vi "HFRR ADV v07.vi"() -> ()   [LabVIEW 2025] (continued)
1.7013246142177483, 1.7065972599989456, 1.7083548085926759, 1.7101123571864059, 1.7136274543738683, 1.7171425515613308, 1.722415197342526, 1.7153850029676008, 1.7101123571864059, 1.7101123571864059, 1.7276878431237184, 1.7171425515613308, 1.7171425515613308, 1.7259302945299884, 1.7259302945299884, 1.741748231873566, 1.7364755860923762, 1.7364755860923762, 1.739990683279836, 1.739990683279836, 1.7382331346861086, 1.7435057804672986, 1.7329604889049162, 1.7329604889049162, 1.7259302945299884, 1.7136274543738683, 1.7101123571864059, 1.7083548085926759, 1.7083548085926759, 1.7083548085926759, 1.7171425515613308, 1.7065972599989456, 1.6960519684365558, 1.6960519684365558, 1.6942944198428282, 1.697809517030288, 1.6960519684365558, 1.6960519684365558, 1.6942944198428282, 1.697809517030288, 1.6925368712490982, 1.6942944198428282, 1.6960519684365558, 1.6890217740616331, 1.6872642254679004, 1.6942944198428282, 1.6837491282804407, 1.6872642254679004, 1.6837491282804407, 1.6802340310929782, 1.6784764824992453, 1.6907793226553656, 1.6855066768741707, 1.6802340310929782, 1.6767189339055155, 1.6749613853117828, 1.6767189339055155, 1.681991579686708, 1.681991579686708, 1.6942944198428282, 1.6890217740616331, 1.6855066768741707, 1.6960519684365558, 1.6925368712490982, 1.6925368712490982, 1.697809517030288, 1.7101123571864059, 1.7083548085926759, 1.7083548085926759, 1.7136274543738683, 1.7189001001550634, 1.7259302945299884, 1.7276878431237184, 1.734718037498646, 1.7329604889049162, 1.7312029403111808, 1.7329604889049162, 1.7382331346861086, 1.734718037498646, 1.7329604889049162, 1.7312029403111808, 1.7329604889049162, 1.734718037498646, 1.739990683279836, 1.7435057804672986, 1.7435057804672986, 1.7470208776547638, 1.7487784262484938, 1.757566169217149, 1.7540510720296862, 1.7558086206234187, 1.771626557966999, 1.7645963635920765, 1.7645963635920765, 1.824353015778937, 1.884109667965795, 1.7997473354666966, 1.7839293981231163, 1.7856869467168466, 1.787444495310579, 1.792717141091774, 1.787444495310579, 1.7804143009356566, 1.782171849529389, 1.7804143009356566, 1.7786567523419266, 1.787444495310579, 1.776899203748194, 1.782171849529389, 1.776899203748194, 1.776899203748194, 1.7804143009356566, 1.787444495310579, 1.792717141091774, 1.7909595924980442, 1.7997473354666966, 1.8050199812478944, 1.8050199812478944, 1.8102926270290869, 1.8120501756228167, 1.8173228214040091, 1.8208379185914743, 1.824353015778937, 1.831383210153857, 1.833140758747592, 1.833140758747592, 1.8366558559350545, 1.8401709531225146, 1.833140758747592, 1.834898307341322, 1.8436860503099772, 1.8366558559350545, 1.8384134045287848, 1.8366558559350545, 1.8384134045287848, 1.8472011474974424, 1.8436860503099772, 1.8507162446849048, 1.8595039876535597, 1.8542313418723673, 1.8612615362472924, 1.866534182028485, 1.8682917306222173, 1.866534182028485, 1.8682917306222173, 1.866534182028485, 1.8682917306222173, 1.8718068278096776, 1.8770794735908725, 1.8700492792159473, 1.8700492792159473, 1.87532192499714, 1.884109667965795, 1.884109667965795, 1.8876247651532576, 1.8893823137469927, 1.8911398623407227, 1.8893823137469927, 1.8946549595281854, 1.898170056715645, 1.898170056715645, 1.8964125081219152, 1.8999276053093779, 1.9016851539031077, 1.9052002510905728, 1.9052002510905728, 1.912230445465498, 1.9069577996843026, 1.9052002510905728, 1.9069577996843026, 1.912230445465498, 1.9052002510905728, 1.9034427024968403, 1.9034427024968403, 1.9016851539031077, 1.9016851539031077, 1.9069577996843026, 1.9104728968717652, 1.912230445465498, 1.9175030912466904, 1.9210181884341528, 1.9210181884341528, 1.913987994059228, 1.9175030912466904, 1.9333210285902707, 1.9227757370278828, 1.9280483828090755, 1.935078577184003, 1.9368361257777331, 1.935078577184003, 1.9473814173401207, 1.945623868746388, 1.9508965145275832, 1.9649569032774308, 1.991320132183401, 1.9596842574962356, 1.9544116117150456, 1.9491389659338532, 1.961441806089971, 1.9561691603087759, 2.049319235776529, 2.0458041385890664, 2.044046589995337, 2.0581069787451844, 2.0686522703075743, 2.0862277562448845, 2.079197561869962, 2.0528343329639918, 1.9825323892147435, 1.970229549058626, 1.9684720004648935, 1.973744646246086, 1.975502194839821, 1.9667144518711634, 1.9684720004648935, 1.975502194839821, 1.973744646246086, 1.973744646246086, 1.973744646246086, 1.973744646246086, 1.973744646246086, 1.971987097652356, 1.9790172920272835, 1.973744646246086, 1.975502194839821, 1.971987097652356, 1.9684720004648935, 1.971987097652356, 1.9667144518711634, 1.9667144518711634, 1.973744646246086, 1.9684720004648935, 1.971987097652356, 1.977259743433551, 1.971987097652356, 1.971987097652356, 1.9983503265583262, 1.977259743433551, 1.9790172920272835, 1.973744646246086, 1.9825323892147435, 1.9807748406210137, 1.9825323892147435, 1.9825323892147435, 1.9860474864022062, 1.977259743433551, 1.9807748406210137, 1.9842899378084762, 1.9842899378084762, 1.9825323892147435, 1.9842899378084762, 1.987805034995936, 1.9842899378084762, 1.9895625835896713, 1.9965927779645936, 1.9930776807771338, 1.9948352293708638, 1.9965927779645936, 2.0001078751520565, 2.0106531667144436, 2.0106531667144436, 2.0141682639019036, 2.017683361089369, 2.024713555464294, 2.026471104058024, 2.0335012984329515, 2.028228652651754, 2.028228652651754, 2.0335012984329515, 2.0352588470266815, 2.0370163956204115, 2.042289041401607, 2.042289041401607, 2.042289041401607, 2.0563494301514544, 2.0475616871827995, 2.0528343329639918, 2.0458041385890664, 2.044046589995337, 2.0458041385890664, 2.049319235776529, 2.0475616871827995, 2.0510767843702618, 2.0545918815577218, 2.0563494301514544, 2.0581069787451844, 2.066894721713842, 2.0616220759326493, 2.0563494301514544, 2.0563494301514544, 2.0510767843702618, 2.0563494301514544, 2.0475616871827995, 2.044046589995337, 2.0458041385890664, 2.044046589995337, 2.0370163956204115, 2.040531492807874, 2.0370163956204115, 2.0335012984329515, 2.0370163956204115, 2.0352588470266815, 2.0299862012454866, 2.0299862012454866, 2.028228652651754, 2.0352588470266815, 2.0352588470266815, 2.073924916088767, 2.135439116869365, 2.0686522703075743, 2.0510767843702618, 2.0475616871827995, 2.049319235776529, 2.0475616871827995, 2.044046589995337, 2.0475616871827995, 2.049319235776529, 2.0510767843702618, 2.0528343329639918, 2.0545918815577218, 2.0581069787451844, 2.049319235776529, 2.049319235776529, 2.0510767843702618, 2.0545918815577218, 2.0545918815577218, 2.0563494301514544, 2.0563494301514544, 2.0616220759326493, 2.066894721713842, 2.0633796245263794, 2.065137173120112, 2.0686522703075743, 2.079197561869962, 2.0827126590574245, 2.0827126590574245, 2.0862277562448845, 2.0932579506198095, 2.0879853048386168, 2.0915004020260795, 2.096773047807272, 2.096773047807272, 2.096773047807272, 2.1055607907759324, 2.103803242182197, 2.1055607907759324, 2.109075887963395, 2.119621179525782, 2.124893825306975, 2.1319240196819003, 2.135439116869365, 2.138954214056825, 2.1442268598380174, 2.14774195702548, 2.153014602806673, 2.153014602806673, 2.1600447971815977, 2.1670749915565253, 2.165317442962793, 2.165317442962793, 2.163559894369063, 2.1670749915565253, 2.1600447971815977, 2.1565296999941355, 2.1547721514004055, 2.153014602806673, 2.1547721514004055, 2.1618023457753304, 2.153014602806673, 2.1582872485878677, 2.1547721514004055, 2.1565296999941355, 2.1582872485878677, 2.1600447971815977, 2.1600447971815977, 2.165317442962793, 2.1705900887439857, 2.1705900887439857, 2.174105185931448, 2.1811353803063755, 2.1758627345251806, 2.1758627345251806, 2.1793778317126433, 2.1758627345251806, 2.1688325401502557, 2.163559894369063, 2.1618023457753304, 2.1565296999941355, 2.1547721514004055, 2.1459844084317505, 2.140711762650558, 2.137196665463095, 2.135439116869365, 2.142469311244288, 2.1336815682756325, 2.1319240196819003, 2.135439116869365, 2.1319240196819003, 2.142469311244288, 2.138954214056825, 2.135439116869365, 2.140711762650558, 2.1442268598380174, 2.1512570542129428, 2.153014602806673, 2.1547721514004055, 2.153014602806673, 2.1547721514004055, 2.195195769056223, 2.1547721514004055, 2.153014602806673, 2.1494995056192128, 2.1459844084317505, 2.1512570542129428, 2.233861838118314, 2.2215589979621937, 2.2268316437433864, 2.233861838118314, 2.2408920324932335, 2.2461646782744262, 2.2619826156180114, 2.2619826156180114, 2.2707703585866668, 2.2408920324932335, 2.2373769353057713, 2.242649581086964, 2.247922226868161, 2.2567099698368165, 2.228589192337116, 2.228589192337116, 2.2461646782744262, 2.1494995056192128, 2.1301664710881676, 2.119621179525782, 2.1161060823383173, 2.112590985150855, 2.1108334365571246, 2.1055607907759324, 2.100288144994735, 2.096773047807272, 2.100288144994735, 2.098530596401002, 2.103803242182197, 2.098530596401002, 2.0932579506198095, 2.1020456935884697, 2.0950154992135395, 2.0950154992135395, 2.0915004020260795, 2.0950154992135395, 2.0915004020260795, 2.103803242182197, 2.0879853048386168, 2.0879853048386168, 2.0844702076511545, 2.079197561869962, 2.077440013276232, 2.0809551104636923, 2.077440013276232, 2.0686522703075743, 2.0721673674950347, 2.0633796245263794, 2.0616220759326493, 2.0528343329639918, 2.0458041385890664, 2.0370163956204115, 2.031743749839216, 2.028228652651754, 2.022956006870561, 2.017683361089369, 2.0088956181207114, 2.0053805209332487, 2.0018654237457887, 2.0001078751520565, 2.0018654237457887, 1.9965927779645936, 1.987805034995936, 1.977259743433551, 1.975502194839821, 1.970229549058626, 1.9579267089025083, 1.9561691603087759, 1.9473814173401207, 1.9403512229651956, 1.9333210285902707, 1.9280483828090755, 1.9192606398404206, 1.9087153482780355, 1.8999276053093779, 1.8999276053093779, 1.884109667965795, 1.8682917306222173, 1.8595039876535597, 1.8454435989037095, 1.834898307341322, 1.8225954671852072, 1.8120501756228167, 1.7979897868729666, 1.7944746896855042, 1.7839293981231163, 1.7751416551544614, 1.7663539121858065, 1.7505359748422236, 1.7470208776547638, 1.7312029403111808, 1.722415197342526, 1.7171425515613308, 1.699567065624018, 1.6855066768741707, 1.6732038367180504, 1.666173642343128, 1.6573858993744703, 1.6468406078120825, 1.6362953162496976, 1.62926512187477, 1.6204773789061149, 1.6134471845311897, 1.6116896359374573, 1.6029018929688048, 1.592356601406417, 1.61520473312492, 1.6837491282804407, 1.7013246142177483, 1.6064169901562673, 1.5695084696879091, 1.5536905323443317, 1.5431452407819417, 1.5431452407819417, 1.5273273034383614, 1.5220546576571663, 1.5273273034383614, 1.523812206250899, 1.523812206250899, 1.5273273034383614, 1.5202971090634363, 1.5325999492195568, 1.5273273034383614, 1.5308424006258214, 1.5431452407819417, 1.544902789375674, 1.5484178865631366, 1.5589631781255242, 1.5695084696879091, 1.5835688584377594, 1.5905990528126872, 1.5976292471876095, 1.6046594415625373, 1.6222349274998475, 1.62926512187477, 1.63981041343716, 1.6591434479682001, 1.6714462881243206, 1.6837491282804407, 1.7030821628114805, 1.7136274543738683, 1.729445391717451, 1.7505359748422236, 1.7663539121858065, 1.7892020439043117, 1.8085350784353542, 1.831383210153857, 1.8524737932786348, 1.8788370221846022, 1.9052002510905728, 1.9315634799965378, 1.961441806089971, 1.987805034995936, 2.026471104058024, 2.0581069787451844, 2.0915004020260795, 2.1284089224944376, 2.1618023457753304, 2.198710866243686, 2.233861838118314, 2.2830731987427813, 2.3270119135860616, 2.379738371398, 2.418404440460088, 2.4711308982720213, 2.532645099052614, 2.5888866540520126, 2.650400854832605, 2.725975444363046, 2.7646415134251336, 2.8243981656119947, 2.9210633382672135, 3.0124558651412365, 3.084515357484215, 3.1706352385770455, 3.262027765451069, 3.3569353895125524, 3.4606307565426935, 3.566083672166567, 3.6662639420092455, 3.7699593090393866, 3.8806848704444525, 3.993167980443254, 4.10213599325459, 4.2111040060659235, 4.3323748590333775, 4.4448579690321735, 4.562613724812167, 4.683884577779619, 4.812185625122, 4.944001769651841, 5.086363205744065, 5.235754836211222, 5.386904015272106, 5.52926545136433, 5.687444824800141, 5.8368364552672976, 5.9967733772968375, 6.30610192979353, 6.478341691979186, 6.643551259789921, 6.808760827600658, 6.965182652442734, 7.137422414628394, 7.29032914228301, 7.492447230562097, 7.636566215248059, 7.747291776653125, 7.900198504307739, 8.067165620712203, 8.197224216648312, 8.429220631020835, 8.585642455862914, 8.749094475079918, 8.949455014765274, 9.075998513513923, 9.239450532730922, 9.40817519772912, 9.559324376790004, 9.675322583976262, 9.866895380692966, 9.9758633935043, 10.13580031553384, 10.293979688969653, 10.429310930686956, 10.59276294990396, 10.649004504903356, 10.823001815682744, 10.90209150240065, 11.049725584274075, 11.228995540834658, 11.366084331145693, 11.508445767237916, 11.642019460361494, 11.768562959110136, 11.905651749421176, 12.065588671450715, 12.241343530823832, 12.371402126759948, 12.585823055195151, 12.606913638319927, 12.867030830192144, 13.185147125657501, 13.396052956905242, 13.603443690965518, 13.83192500815058, 14.789788991734092, 17.011330414210352, 16.030618298908333, 15.981406938283856, 16.07455701375161, 15.802136981723274, 15.800379433129542, 16.00425507000236, 16.248554324531, 16.299523233749206, 16.77757645124409, 17.11151068405303, 16.812727423118723, 17.187085273583474, 16.94630111624229, 17.89713490545088, 18.072889764823994, 17.842650899045214, 17.6563507481097, 17.695016817171783, 17.872529225138642, 17.911195294200724, 17.890104711075956, 18.043011438730566, 17.958649106231476, 18.048284084511764, 18.072889764823994, 18.004345369668485, 18.148464354354438, 18.1801002290416, 18.17131248607295, 18.25040217279085, 18.257432367165777, 18.31367392216517, 18.35058244263353, 18.403308900445467, 18.41561174060159, 18.392763608883076, 18.459550455444862, 18.4841561357571, 18.507004267475608, 18.51930710763173, 18.57203356544366, 18.58960905138097, 18.619487377474403, 18.642335509192907, 18.64936570356783, 18.60718453731829, 18.605426988724552, 18.59839679434963, 18.57730621122485, 18.59488169716217, 18.56500337106873, 18.55797317669381, 18.57027601684993, 18.56676091966247, 18.531609947787846, 18.538640142162766, 18.528094850600382, 18.521064656225455, 18.52985239919411, 18.5122769132568, 18.482398587163367, 18.605426988724552, 18.614214731693213, 18.56148827388127, 18.56500337106873, 18.57203356544366, 18.549185433725157, 18.540397690756503, 18.52985239919411, 18.52985239919411, 18.5122769132568, 18.51403446185053, 18.515792010444265, 18.482398587163367, 18.494701427319487, 18.475368392788447, 18.464823101226052, 18.443732518101285, 18.459550455444862, 18.44900516388247, 18.427914580757704, 18.45076271247621, 18.436702323726358, 18.42439948357024, 18.433187226538898, 18.427914580757704, 18.408581546226657, 18.41385419200785, 18.389248511695616, 18.398036254664273, 18.38573341450815, 18.38221831732069, 18.38221831732069, 18.35058244263353, 18.368157928570838, 18.348824894039797, 18.34706734544607, 18.340037151071144, 18.331249408102487, 18.327734310915027, 18.31543147075891, 18.31543147075891, 18.301371082009055, 18.287310693259204, 18.297855984821588, 18.280280498884274, 18.275007853103087, 18.269735207321887, 18.25567481857205, 18.252159721384576, 18.232826686853535, 18.239856881228466, 18.215251200916224, 18.217008749509954, 18.209978555135034, 18.19064552060399, 18.195918166385184, 18.183615326229067, 18.169554937479216, 18.17307003466668, 18.153737000135635, 18.151979451541898, 18.137919062792054, 18.125616222635934, 18.12737377122967, 18.115070931073546, 18.115070931073546, 18.10276809091743, 18.099252993729966, 18.095737896542506, 18.09046525076131, 18.081677507792655, 18.067617119042804, 18.062344473261614, 18.055314278886687, 18.044768987324296, 18.03598124435564, 18.032466147168176, 18.023678404199522, 18.025435952793252, 18.021920855605796, 18.00961801544967, 17.99907272388729, 17.997315175293558, 17.99204252951236, 17.98501233513744, 17.97095194638759, 17.963921752012663, 17.958649106231476, 17.953376460450276, 17.946346266075352, 17.934043425919235, 17.93580097451296, 17.97095194638759, 17.953376460450276, 17.955134009044006, 17.94283116888789, 17.93931607170043, 17.927013231544308, 17.921740585763114, 17.891862259669683, 17.895377356857146, 17.89889245404461, 17.893619808263416, 17.881316968107296, 17.88307451670103, 17.879559419513566, 17.865499030763715, 17.833863156076553, 17.837378253264013, 17.80925747576432, 17.796954635608202, 17.796954635608202, 17.78465179545208, 17.77234895529596, 17.767076309514763, 17.777621601077154, 17.774106503889694, 17.742470629202533, 17.768833858108493, 17.719622497484025, 17.724895143265222, 17.724895143265222, 17.7178649488903, 17.728410240452682, 17.707319657327908, 17.70028946295298, 17.716107400296565, 17.703804560140444, 17.677441331234476, 17.65107810232851, 17.66865358826582, 17.5772610613918, 17.53859499232971, 17.52277705498613, 17.52453460357986, 17.515746860611202, 17.51047421483001, 17.50871666623628, 17.49992892326762, 17.491141180298964, 17.480595888736577, 17.477080791549124, 17.466535499986733, 17.464777951393007, 17.45423265983061, 17.44720246545569, 17.43314207670584, 17.43489962529957, 17.43138452811211, 17.419081687955984, 17.4085363963936, 17.403263750612407, 17.403263750612407, 17.390960910456286, 17.38744581326883, 17.382173167487633, 17.368112778737785, 17.368112778737785, 17.35405238998793, 17.347022195613008, 17.34174954983182, 17.339992001238087, 17.329446709675697, 17.325931612488237, 17.31714386951958, 17.308356126550922, 17.304841029363462, 17.303083480769722, 17.29429573780107, 17.278477800457495, 17.2732051546763, 17.26969005748884, 17.26265986311391, 17.257387217332717, 17.252114571551527, 17.245084377176603, 17.239811731395402, 17.23805418280167, 17.223993794051825, 17.223993794051825, 17.22047869686436, 17.213448502489445, 17.209933405301975, 17.20290321092705, 17.192357919364667, 17.188842822177204, 17.178297530614817, 17.17478243342735, 17.15720694749004, 17.146661655927648, 17.14490410733392, 17.136116364365265, 17.12908616999034, 17.122055975615414, 17.113268232646764, 17.178297530614817, 17.162479593271232, 17.115025781240494, 17.08338990655333, 17.081632357959595, 17.081632357959595, 17.067571969209745, 17.067571969209745, 17.06054177483482, 17.05702667764736, 17.051754031866164, 17.042966288897507, 17.035936094522594, 17.02363325436647, 17.01484551139781, 17.00957286561662, 16.995512476866768, 16.991997379679308, 16.990239831085574, 16.98496718530438, 16.979694539523184, 16.977936990929454, 16.96387660217961, 16.95508885921095, 16.951573762023486, 16.94278601905482, 16.933998276086164, 16.933998276086164, 16.92169543593005, 16.91642279014886, 16.9129076929614, 16.91642279014886, 16.904119949992744, 16.897089755617817, 16.895332207024087, 16.88654446405543, 16.87775672108677, 16.883029366867966, 16.867211429524385, 16.858423686555728, 16.85490858936826, 16.846120846399604, 16.832060457649764, 16.83030290905603, 16.823272714681107, 16.81624252030618, 16.810969874524982, 16.802182131556325, 16.8004245829626, 16.789879291400208, 16.789879291400208, 16.781091548431554, 16.768788708275437, 16.770546256869167, 16.767031159681704, 16.756485868119317, 16.754728319525583, 16.745940576556933, 16.738910382182006, 16.733637736400812, 16.724849993432162, 16.716062250463505, 16.702001861713647, 16.69672921593246, 16.698486764526187, 16.684426375776336, 16.682668827182606, 16.677396181401413, 16.666850889839022, 16.661578244057836, 16.659820695464106, 16.64927540390171, 16.640487660933058, 16.633457466558134, 16.628184820776944, 16.622912174995744, 16.622912174995744, 16.615881980620824, 16.60533668905843, 16.600064043277243, 16.59830649468351, 16.5807310087462, 16.577215911558728, 16.573700814371275]
  in  "ENTER THE NEW PASSWORD":string caption="Enter The New Password"
  in  "ENTER CURRENT PASSWORD":string caption="Enter Current Password"
  in  "Camera Port :":string(combo)="cam0"
  in  "Humidity :":refnum<visa-resource-name>="COM8"
  in  "LvdtOff":dbl=2.875 caption="LVDT Position Offset :" min=2.1 max=2.9 format="%.4f"
  out "Port 2 Error":errorcluster={"status"=TRUE, "code"=-1073807343, "source"="Property Node (arg 1) in VISA Configure Serial Port (Instr).vi->Winducom 2010--std ed hfrr-wo1768-V18.vi"}
  out "Port 1 Error":errorcluster={"status"=TRUE, "code"=-1073807343, "source"="Property Node (arg 1) in VISA Configure Serial Port (Instr).vi->Winducom 2010--std ed hfrr-wo1768-V18.vi"}
  in  "Stroke PID Gains":T9={"Proportional Gain (Kc)"=200.0, "Integral Time (Ti, min)"=0.02, "Derivative Time (Td, min)"=0.0}
  in  "CH-HUMIDITY DRY":u16=3 caption="Ch-Humidity Wet:" max=7 step=1
  in  "CH-HUMIDITY WET":u16=4 caption="Ch-Humidity Dry:" max=7 step=1
  in  "CH-HEATER":u16=2 caption="Ch-Heater:" max=7 step=1
  in  "CH-POWER -":u16=1 caption="Ch-Power -:" max=7 step=1
  in  "CH-POWER +":u16 caption="Ch-Power +:" max=7 step=1
  out "String 4":string
  in  "Prog Due":bool
  in  "Prog Uno":bool
  in  "Com Port 2":refnum<visa-resource-name>="COM7" caption="Port 2 :"
  in  "Com Port 1":refnum<visa-resource-name>="COM5" caption="Port 1 :"
  in  "Tab Control 6":enum32{"Data", "Sensor"}(tab)=enum."Sensor"
  out "Respose From Server":string
  out "standard output":string
  out "SinglePoint":string
  in  "JSON Check String":string="\"Stored\": true"
  in  "JSONH Check String":string="\"Stored\": true"
  out "standard output 2":string
  in  "Sensor Information":string[][](array[string])=[["Sensor Name", "Sensor Model Number", "Sensor Run time Hours", "Sensor State"], ["Normal Load Sensor", "MPF-AC20-X3U791", "", ""], ["Frictional Force Sensor", "MPF-AC20-X3U792", "", ""], ["Temperature Sensor", "MPF-AC20-X3U793", "", ""], ["Speed Sensor", "MPF-AC20-X3U794", "", ""], ["LVDT Sensor", "MPF-AC20-X3U795", "", ""], ["Vibration Sensor ", "MPF-AC20-X3U796", "", ""]]
  out "Respose From Server 2":string
  in  "Total No. of Tests":dbl
  in  "Upld AR":bool
  in  "Sensor File Name":string="JSON_Health.JSON"
  in  "Run test 3":bool
  in  "Sen.Upload Rate (s)":dbl=5.0 min=0.5 max=5.0 step=0.5 format="%.1g"
  in  "Upld AR 2":bool
  in  "Path":path=path "C:/LAB-IQ-NXT"
  in  "Data File Name":string="JSON_Single_Point.JSON"
  in  "Model No":string="MD987654325"
  in  "Serial No":string="HFRR2391"
  in  "Secret Key":string="22gKHnAGFaJhuNtaR9srYhcD6RQR8M7Zp2xk4ssPTuwGqWUBv7WxW7cXAFkFFbns"
  in  "Upload Rate (s)":dbl=1.0 min=0.5 max=5.0 step=0.5 format="%.1g"
  in  "STOP 2":bool
  in  "service 2":bool caption="Password"
  in  "ADC Res":u16(ring) items=["16 bit", "24 bit"]
  out "Test Standard":string
  out "error out 5":errorcluster
  out "after substring":string
  out "before substring 2":string
  in  "Temperature after test 3":dbl caption="Temp After Test" format="%#_5g"
  in  "Humidity after test 3":dbl caption="Humidity After Test" format="%#_5g"
  in  "Tab Control 4":T10(tab)=enum."Temperature Tuning"
  in  "ECR_Gain":dbl=24000.0
  out "Ch3 2":dbl[](graph)
  out "Air temp":dbl[](graph)
  out "ECR":dbl[](graph)
  out "Rtemp":dbl[](graph)
  in  "Do 0":bool
  out "DI 0":bool=TRUE
  out "DI 1":bool=TRUE
  out "DI 2":bool=TRUE
  out "DI 3":bool=TRUE
  out "DI 4":bool=TRUE
  out "DI 5":bool=TRUE
  out "DI 6":bool=TRUE
  out "DI 7":bool=TRUE
  in  "Do 7":bool
  in  "Do 6":bool
  in  "Do 5":bool
  in  "Do 4":bool
  in  "Do 3":bool
  in  "Do 2":bool
  in  "Do 1":bool
  in  "output range":cluster{"output high":dbl, "output low":dbl}={"output high"=110.0, "output low"=0.0}
  in  "Offset Air Temp":dbl
  in  "Temp PID gains":T11={"proportional gain (Kc)"=10.0, "integral time (Ti, min)"=1.66, "derivative time (Td, min)"=0.0}
  out "gTEMP 3":cluster{dbl, "output":dbl, "Set Temp":dbl}(graph)={6.858462627117447, "output"=42.16277107130474, "Set Temp"=53.14153737288255}
  out "Pk-Pk":dbl=0.5
  in  "Offset":dbl=0.5
  in  "Gain":dbl=1.4
  out "gLVDTraw":dbl[](graph)
  out "Disp":dbl=-1.7485910993892546e-16 caption="Stroke" format="%.2f"
  out "Freq":dbl=50.0 caption="Frequency" min=10.0 max=250.0 step=0.1 format="%.2f"
  out "PID Out":u8(slide) scale=0.0..4095.0
  out "Freq":dbl min=0.0 max=12.0 step=0.01 format="%.3f"
  out "Array":string[](array[string])
  out "UnoRead":string
  out "Sps 2":dbl=890.0 format="%_0f"
  out "Disp (mm)":dbl=1.0 min=0.0 max=12.0 step=0.01 format="%.3f"
  in  "PID Rst":bool=TRUE
  in  "DC correction":bool=TRUE
  out "Mean(RAW) Stroke":dbl(graph)
  out "Waveform Graph 2":waveform(dbl)[](graph)
  in  "Tab Control 8":enum32{"setup", "calibrate"}(tab)
  in  "Boolean 10":bool
  in  "Measure":bool
  in  "Measure 2":bool
  in  "Boolean 11":bool
  in  "Zero 4":bool
  out "Intercept":dbl
  out "Slope":dbl
  in  "Captured Values 2":dbl[][](array[numeric])
  in  "Zero 3":bool
  out "software msrnt":dbl=50.0 caption="Software measurment" min=0.0 max=250.0 step=0.001 format="%.4f"
  out "Measure_LDS":dbl=50.0 caption="Position (high precision laser)" min=0.0 max=250.0 step=0.001 format="%.4f"
  in  "Boolean 9":bool
  in  "Boolean 8":bool
  in  "Boolean 7":bool
  out "?":cluster{"Y":dbl[], "Y":dbl[]}[](graph)
  in  "Laser Disp Sensor":refnum<visa-resource-name>="COM14" caption="COM Port"
  in  "COMMAND":string="OUTPUT RS422"
  in  "COMMAND 2":string="OUTPUT NONE\n"
  in  "ACQUIRE 2":bool
  out "Friction Force (N)":ext=1.0 format="%_4f"
  out "G_val":dbl
  out "Current (A)":ext=1.0 format="%_4f"
  in  "Window":ext=1.0
  out "Constant (G)":dbl(graph)
  out "Waveform Graph 4":dbl[][](graph)
  in  "Humidity BaudRate":dbl=9600.0
  in  "Re-Initialise":bool
  out "Humidity 2":u32(graph)
  out "Port 2":u32(graph)
  out "Port 1":u32(graph)
  out "autostrtflg":bool
  out "airtempflg":bool
  out "z_measure":dbl
  in  "ACQUIRE 3":bool
  out "pk-pk":cluster{dbl, "t":dbl}(graph)
  out "Read String":string
  out "Waveform Graph 5":dbl[](graph)
  out "Waveform Chart 3":dbl[](graph)
  out "set temp old":dbl
  out "Error Code":errorcluster
  in  "Rd":bool
  out "String 10":string
  in  "Length 2":i16=16 caption="Set" min=1 max=60 step=1
  out "path 2":path
  out "image data":T12
  out "new picture":picture
  out "error out 2":errorcluster
  out "String Indicator 4":string
  out "String Indicator 3":string
  in  "OPEN 5":bool
  out "string1 5":string
  out "String 49":string="Tested by"
  out "String 48":string="Sample ID "
  out "String 47":string="Tested date"
  out "String 46":string="S.NO"
  out "test by 2":string
  in  "ISO : WS1.4":enum32{"Page 1", "Page 2"}(tab)
  in  "Save Results":bool
  out "String 23":string="ISO : WS1.4"
  out "Rh After":dbl min=0.0 max=100.0 step=1.0 format="%.1f"
  out "Rh Before":dbl min=0.0 max=100.0 step=1.0 format="%.1f"
  in  "Humidity before test":dbl min=0.0 max=100.0 step=1.0
  out "AVP":dbl=0.0032746494993313616 format="%.3f"
  in  "MWSD":dbl
  out "WS1.4":dbl format="%1.2f"
  in  "HCF":dbl min=0.0 max=10000.0 step=0.01 format="%.2f"
  in  "Temperature before test":dbl=1.0 caption="Temp before test" min=1.0 max=100.0 step=0.1 format="%.1f"
  in  "Humidity after test":dbl=1.0 min=1.0 max=100.0 step=1.0
  in  "Temperature after test":dbl=1.0 caption="Temp after test" min=1.0 max=100.0 step=0.1 format="%.1f"
  out "WS1.4 2":dbl caption="WS1.4" format="%#_5g"
  out "HCF 2":dbl caption="HCF" format="%#_5g"
  out "AVP 2":dbl caption="AVP" format="%#_5g"
  out "MWSD 2":dbl caption="MWSD" format="%#_5g"
  out "Temperature after test 2":dbl caption="Temp after test" format="%#_5g"
  out "Humidity after test 2":dbl caption="Humidity after test" format="%#_5g"
  out "Temperature before test 2":dbl caption="Temp before test" format="%#_5g"
  out "Humidity before test 2":dbl caption="Humidity before test" format="%#_5g"
  out "Voltage LVDT Acq":dbl[](graph)
  out "Stroke_send_Val":string
  out "AirT":dbl(graph)
  out "temp_@Rh sensor":string
  out "refresh flag":bool
  out "Air temp":string
  in  "hide controller":enum32{"Hidden", "controllers"}(tab)=enum."controllers"
  in  "UUID":string caption="UUID    :"
  in  "FLAG 4":dbl min=0.0 max=999999999.0 step=0.25 format="%.2f"
  out "START 3":dbl format="%.1f"
  in  "FLAG 2":dbl min=0.0 max=999999999.0 step=0.25 format="%.2f"
  out "JSON string":string
  out "Sensor Health JSON string":string
  out "run replace":bool
  out "cof":dbl caption="Frictional Torque" format="%.2f"
  out "time":dbl caption="Time \nRemaining"
  out "SEN.RUN HRS":dbl
  out "Json St Flg":bool
  out "Json End Flg":bool
  out "temp_st":string
  out "sp_st":string
  out "FF STATE":i32
  out "nlstate":string
  out "ffstate":string
  out "nl_st":string
  out "ff_st":string
  in  "in":string[](array[string])=["", "", "", "", "", "", ""]
  out "out":string[](array[string])=["Sensor State", "", "", "", "", "", ""]
  out "SinglePoint  2":string
  out "Sensor name":string[](array[string])
  out "model num":string[](array[string])
  out "run time":string[](array[string])
  out "state":string[](array[string])
  out "state1":string[](array[string])
  out "T cycle":dbl caption="TOTAL\nTIME"
  in  "Length":i16=16 caption="Set" min=1 max=60 step=1
  out "acq 2":bool
  out "Stroke Ln 2":string
  out "St Str":string
  out "run":string[](array[string])
  out "ecr 2":dbl caption="Pin temp"
  out "run hrs":string
  in  "tfalg":dbl
  out "Temp":dbl caption="Pin temp"
  in  "yflag":dbl
  in  "zflag":dbl
  out "zflag 2":dbl
  out "Stroke Ln":dbl caption="Normal Load"
  out "SENSOR TIME":dbl
  out "TEMP STATE":i32
  out "NL STATE":i32
  in  "FLAG":dbl min=0.0 max=999999999.0 step=0.25 format="%.2f"
  out "START 2":dbl format="%.1f"
  out "SENSOR TIME  2":dbl
  out "Rt 3":bool
  out "Rt":bool
  out "Rt 2":bool=TRUE
  out "Elapsed time":dbl caption="Elapsed Time" min=0.0 max=6000.0 step=0.01 format="%.2f"
  in  "Reset 4":bool caption="Reset"
  in  "tmpchk":bool
  out "Temp ini":dbl min=0.0 max=150.0 step=1.0
  in  "wait":u32=1000
  out "humid":string
  out "Ser Led":bool
  in  "Send":bool
  out "Humidity Str Rec":string
  in  "Humidity Str Send":string="stop"
  out "String 9":string
  in  "Reset 3":bool caption="Reset"
  in  "check time s":dbl=10.0
  in  "Threshold value":dbl=1000.0
  out "file count":i32
  out "Waveform Graph":dbl[][](graph)
  in  "Hold 4":bool
  in  "save dpt":bool
  in  "FILE 2":string="Spike Cpture" caption="File name"
  out "Humid Last buf":dbl[](graph)
  out "visa due":string(combo)="COM63" caption="Visa Module 2 ( Due )"
  in  "Tab Control":T13(tab)
  out "String 43":string="mm"
  in  "Home 8":bool
  in  "Home 9":bool
  out "String 18":string="min"
  out "String 22":string="min"
  out "String 17":string="Timer"
  in  "Samplingtime 2":dbl=0.5 caption="Save Dwell" min=0.1 max=600.0 step=0.1 format="%.1g"
  out "String 21":string="Sec"
  in  "RST FF":bool
  in  "RSTCOF 3":bool
  in  "RST TEMP":bool
  in  "RSTCOF":bool
  in  "Home":bool caption="Password"
  in  "Configure":bool caption="Password"
  in  "Analysis 2":bool caption="Password"
  in  "service 3":bool caption="Password"
  in  "EXIT 2":bool
  in  "GRAY SCALE INTERCHANGE":enum32{"GRAY IMAGE", "RGB IMAGE"}(radio)=enum."RGB IMAGE"
  in  "Lubrication System COM Port :":refnum<visa-resource-name>="COM9" caption="Ambient Temperature COM Port:"
  in  "Com Port 3":refnum<visa-resource-name>="COM4" caption="Port 3"
  in  "autostart":bool caption="RUN"
  in  "SetTemp 2":dbl=23.0 caption="Set" min=1.0 max=26.0 step=1.0
  out "autostart 2":string
  out "String 14":string
  out "TK4 status":bool=TRUE caption="Air Status"
  in  "Heater":bool
  out "Amb temp":dbl caption="Air Temperature" min=0.0 max=150.0 step=1.0 format="%.1f"
  out "SetTemp":dbl=23.0 caption="Set" min=20.0 max=26.0 step=1.0
  in  "Engage":bool
  out "Countdown 2":dbl caption="Present ( Sec )" min=1.0 max=6000.0 step=1.0
  in  "Countdown":dbl=1.0 caption="Count down ( Sec )" min=1.0 max=6000.0 step=1.0
  in  "PWR":bool
  in  "st enable":bool
  out "COF - filtered":dbl min=0.0 max=200.0 step=0.1 format="%.2f"
  in  "% Humidity":dbl=35.0 min=1.0 max=100.0 step=1.0
  out "Peak - Peak 2":dbl
  out "COF":dbl=100.0 min=0.0 max=200.0 step=0.1 format="%.1f"
  out "act save time":dbl=3561152582.7339997 format="%.2f"
  out "acq timer":dbl=3614575087.823 format="%.2f"
  out "Cycles elapsed":i32=5
  in  "Save":bool
  out "cyclecount":i32
  out "speedop":dbl min=0.0 max=999999999.0 step=0.25 format="%.2f"
  out "cmp":i32
  in  "OPEN 6":bool
  out "freq1":dbl format="%_4f"
  out "freq2":dbl format="%_4f"
  out "freq3":dbl format="%_4f"
  out "sample1":dbl format="%_4f"
  out "sample2":dbl format="%_4f"
  out "sample3":dbl format="%_4f"
  out "String 6":string="  "
  in  "String 7":string="  "
  out "String 12":string="  "
  out "String 8":string="  "
  out "Numeric 13":i32
  out "Numeric 12":i32
  out "Numeric 11":i32
  out "Numeric 8":i32
  in  "Ref B Scar Value :":string caption="Reference Fluid Information"
  in  "Ref B Test Date :":string caption="Reference Fluid Information"
  in  "Ref A Scar Value :":string caption="Reference Fluid Information"
  in  "Image Path":path
  in  "Wear Scar Y":dbl caption="Wear Scar Minor Axis ( Microns )" format="%#_5g"
  in  "Wear Scar X":dbl caption="Wear Scar Major Axis ( Microns )" format="%#_5g"
  in  "Print 2":bool caption="Печать"
  in  "Ref A Test Date :":string caption="Reference Fluid Information"
  out "XY Graph 17":cluster{dbl[], dbl[]}[](graph)
  in  "Print 3":bool caption="Печать"
  in  "Select File Type":enum16{"xlx", "csv", "txt"}(ring)
  out "s.NO":string caption="S.NO"
  in  "Export":bool
  out "Test Date":string caption="Tested date"
  out "Tested by":string
  out "Sample ID":string
  in  "OK Button 16":bool
  out "String Indicator":string
  out "String Indicator 2":string
  in  "OK Button 17":bool
  out "Selected Printer":string="Microsoft XPS Document Writer"
  in  "Select Printer 3":i32 caption="Select Printer"
  out "System Configured Printers 2":string[](array[string])=["Microsoft XPS Document Writer", "Fax", "CutePDF Writer", "\\\\192.168.1.28\\RICOH Aficio MP 2352 PCL 6"] caption="System Configured Printers"
  out "TITTLE":string caption="Tittle"
  in  "Sample ID  5":string caption="Fuel S/N:"
  in  "Sample ID  4":string caption="Fuel Name:"
  in  "Sample ID  3":string caption="Fuel Type:"
  in  "Print":bool caption="Печать"
  in  "message":string="*Entered password is wrong"
  in  "SPEED OUT:":dbl=1.0 caption="Speed Out:" min=0.0001 max=5.0 step=0.0001 format="%.4f"
  in  "Temperature before test 3":dbl caption="Temp Before Test" format="%#_5g"
  in  "Humidity before test 3":dbl caption="Humidity Before Test" format="%#_5g"
  out "Temperature after test 5":dbl caption="Temp Before Test" format="%#_5g"
  out "Temperature after test 4":dbl caption="Temp After Test" format="%#_5g"
  out "Humidity after test 4":dbl caption="Humidity After Test ( % Rh )" format="%#_5g"
  out "Humidity before test 4":dbl caption="Humidity Before Test ( % Rh )" format="%#_5g"
  in  "Tab Control 9":enum32{"Page 1", "Page 2"}(tab)
  out "Ref B Scar Value :":string caption="Reference Fluid Information"
  out "Ref B Test Date :":string caption="Reference Fluid Information"
  out "Ref A Scar Value :":string caption="Reference Fluid Information"
  out "Ref A Test Date :":string caption="Reference Fluid Information"
  out "XY Graph 16":cluster{dbl[], dbl[]}[](graph)
  out "TITTLE 4":string caption="Reference Fluid Information"
  out "Sample ID  7":string caption="Fuel Name :"
  out "Sample ID  6":string caption="Fuel Type :"
  out "Mean Wear ( microns) :":dbl format="%#.6f"
  out "Wear Scar Y ( microns ) :":dbl format="%#.6f"
  out "Length ( microns ) 2":dbl caption="Wear Scar X ( microns ) :" format="%#.6f"
  out "s.NO 2":string caption="Instrument  S.NO :"
  out "Test Date 2":string caption="Tested date :"
  out "Tested by 2":string caption="Tested by :"
  out "Sample ID  2":string caption="Sample ID :"
  out "TITTLE 2":string caption="File Name :"
  in  "EDIT 3":bool
  out "FF buffer":dbl[](graph)
  out "%  o/p":dbl
  out "sample4":dbl format="%_4f"
  out "freq 4":dbl format="%_4f"
  out "conststatus":dbl=10.0 min=0.0 max=200.0 step=1.0
  out "CP4":dbl=nan min=0.0 max=200.0 step=0.1 format="%.3f"
  out "CP3":dbl=nan min=0.0 max=200.0 step=0.1 format="%.3f"
  out "Boolean  4":bool=TRUE caption="Power Status"
  in  "Boolean BC T & BG 2":cluster{u32, u32}[](array[cluster])=[{3158064, 16250871}, {11918296, 8965631}]
  in  "GBG   2":u32(colorbox)=16250871 caption="Graph Background"
  in  "GFG  2":u32(colorbox)=8964095 caption="Graph Foreground"
  in  "GBG":u32(colorbox)=16250871 caption="Graph Background"
  in  "GFG":u32(colorbox)=8964095 caption="Graph Foreground"
  in  "Boolean BC T & BG":cluster{u32, u32}[](array[cluster])=[{3158064, 16250871}, {11918296, 8965631}]
  in  "SC  Text":u32(colorbox) caption="String Control Text"
  in  "SC BG 3":u32(colorbox)=16777215 caption="String Control BG"
  in  "NI BG 2":u32(colorbox)=13553358 caption="Numeric Indicator BG"
  in  "NI Text  2":u32(colorbox)=7105644 caption="Numeric Indicator Text"
  in  "NC Text":u32(colorbox)=3381759 caption="Numeric Control Text"
  in  "NC BG":u32(colorbox)=16777215 caption="Numeric Control BG"
  out "ABS DP":dbl[](graph)
  in  "Com flag":u32
  out "Gain path":string="C:\\Winducom 2010\\STD ED HFRR\\wo1768"
  out "String 45":string="S.NO"
  out "String 44":string
  out "error out 4":errorcluster
  out "concatenated string 2":string
  out "String 42":string
  out "error out 3":errorcluster
  out "STR":string
  out "gain":string
  out "export":string
  out "before substring":string
  out "output":string
  out "test by":string
  out "export 2":string
  out "export":string
  out "REMARKS 2":string="@WINDUCOM : RECIPROCATORY TEST RIG    DEFINITON FILE       \r  Sample ID :- , Load :-  2.00 N , Remarks :- , Date :- 05/11/2016, 06:04\r"
  out "data":string
  out "Boolean 3":bool
  out "String 41":string=":-@(WINDUCOM : RECIPROCATORY TEST RIG    DEFINITON FILE )      "
  out "concatenated string":string
  out "path":path
  out "String 40":string
  out "Boolean 2":bool=TRUE
  in  "Set Rh 2":dbl=50.0 caption="HUMIDITY" min=35.0 max=85.0 step=1.0
  out "String 39":string="WS1.4="
  out "String 38":string="HCF="
  out "String 37":string="MWSD="
  out "String 36":string="AVP ="
  out "String 35":string="Temp after test="
  out "String 34":string="Temp before test="
  out "String 33":string="Tested by"
  out "String 32":string="Sample ID "
  out "String 31":string="Tested date"
  out "String 30":string="Sample Design"
  out "path string":string
  out "String 29":string
  out "St. Line eqn : 2":string
  out "Numeric 10":i32
  out "Numeric 16":i32
  out "S 106":string="Off"
  out "S 105":string="On"
  out "S 104":string="Heater Off"
  out "S 103":string="Heater On"
  out "S 102":string="Ch-Humidity Dry:"
  out "S 101":string="Ch-Humidity Wet:"
  out "S 100":string="Ch-Heater:"
  out "S 99":string="Ch-Power -:"
  out "S 98":string="Ch-Power +:"
  out "S 97":string="Port 2"
  out "S 96":string="Port 1"
  out "S 95":string="Stroke Gain :"
  out "S 94":string="Displacement :"
  out "S 93":string="Stop"
  out "S 92":string="Run"
  in  "LAnguage":enum32{"Page 1", "Page 2"}(tab)
  out "S 91":string="Threshold"
  out "S 90":string="File path"
  out "S 89":string="Newtons ( N )"
  out "S 88":string="Change Calibrate Password"
  out "S 87":string="Enter The New Password"
  out "S 86":string="Enter Current Password"
  out "S 85":string="Password"
  out "S 84":string="Save Gain Constants"
  out "S 83":string="Air Temperature ( deg C )"
  out "S 82":string="TIME ( mins )"
  out "S 81":string="Relative Humidity ( Rh )"
  out "S 80":string="Sample TEMPERATURE ( Deg C)"
  out "S 79":string="Stroke"
  out "S 78":string="Air Temperature"
  out "S 77":string="mm"
  out "S 76":string="Stroke"
  out "S 75":string="WINDUCOM 2010 \\XXXX\\VX.XX\\MONTH YEAR"
  out "S 74":string="Frictional Force ( N )"
  out "S 73":string="Calibrate Parameter"
  out "S 72":string="Save Gain Constant"
  out "S 71":string="Edit Gain Constant"
  out "S 70":string="Humidity :"
  out "S 69":string="Air Temperature :"
  out "S 68":string="Speed Out:"
  out "S 67":string="Temperature :"
  out "S 66":string="Frictional Force :"
  out "S 65":string="ABOUT"
  out "S 64":string="Frictional  Force ( N )"
  out "S 63":string="Temperature ( Deg C)"
  out "S 62":string="Time ( mins )"
  out "S 60":string="Reset Graph"
  out "S 59":string="COF4"
  out "S 58":string="COF3"
  out "S 57":string="COF2"
  out "S 56":string="COF1"
  out "S 55":string="Frictional Force ( N )"
  out "S 54":string="Temperature"
  out "S 53":string="Coefficient Of Friction"
  out "S 52":string="Refresh"
  out "S 51":string="File 4"
  out "S 50":string="File 3"
  out "S 49":string="File 2"
  out "S 48":string="File 1"
  out "S 47":string="COMPARE FILES"
  out "S 46":string="SAVE RESULT"
  out "S 45":string="WS1.4"
  out "S 44":string="HCF"
  out "S 43":string="MWSD"
  out "S 42":string="AVP "
  out "S 41":string
  out "S 40":string
  out "S 39":string="Humidity after test="
  out "S 38":string="Humidity before test="
  out "S 37":string
  out "S 36":string="Rh Before"
  out "S 35":string="ISO : WS1.4"
  out "S 34":string="FRICTIONAL FORCE ( N )"
  out "S 33":string="Reset Graph"
  out "S 32":string="Data points"
  out "S 31":string="COEFFICIENT OF FRICTION"
  out "S 30":string="RUN"
  out "S 29":string="Test Status"
  out "S 28":string="Power"
  out "S 27":string="Engage"
  out "S 26":string="Present ( Sec )"
  out "S 25":string="Count down ( sec )"
  out "S 24":string="Sec"
  out "S 23":string="Save Dwell"
  out "S 22":string="Elapsed Time"
  out "S 21":string="min"
  out "S 20":string="Test duration"
  out "S 19":string="TIMER"
  out "S 18":string="OFF"
  out "S 17":string="Rh"
  out "S 16":string="HUMIDITY"
  out "S 15":string="Heater On"
  out "S 14":string="TEMPERATURE ( Deg C)"
  out "S 13":string="N"
  out "S 12":string="NORMAL LOAD"
  out "S 11":string="Hz"
  out "S 10":string="FREQUENCY"
  out "S 9":string="STOP"
  out "S 8":string="STAND BY"
  out "S 7":string="Remarks :"
  out "S 6":string="Sample ID :"
  out "S 5":string="File Name :"
  out "S 4":string="Acquire"
  out "S 3":string="EXIT"
  out "S 2":string="Winducom 2010"
  out "S":string="ENGLISH TITLES"
  out "Error Due":errorcluster={"status"=TRUE, "code"=-1073807343, "source"="Property Node (arg 1) in VISA Configure Serial Port (Instr).vi->Winducom 2010--std ed hfrr-wo1768-V18.vi"}
  out "Error Uno":errorcluster={"status"=TRUE, "code"=-1073807343, "source"="Property Node (arg 1) in VISA Configure Serial Port (Instr).vi->Winducom 2010--std ed hfrr-wo1768-V18.vi"}
  out "as":string
  out "bs":string="Rh After"
  out "as":string=" after test"
  out "bs":string="Temp"
  out "as":string=" before test"
  out "bs":string="Temp"
  out "as":string=" after test"
  out "bs":string
  out "bs":string="Humidity"
  out "as":string=" before test"
  out "bs":string="Humidity"
  out "S 61":string="Frictional Force ( N )"
  in  "Lan flag":dbl=22.0
  in  "Table":string[][](table)=[["ENGLISH TITLES", "RUSSIAN"], ["Winducom 2010", "Winducom  2010"], ["Exit", "Выход"], ["Acquire", "ИСПЫТАНИЕ     "], ["File Name :", "Имя файла :"], ["Sample ID :", "Имя образца :"], ["Remarks :", "Примечания :"], ["Standby", "ОЖИДАНИЕ"], ["Stop", "СТОП"], ["Frequency", "ЧАСТОТА"], ["Hz", "Гц"], ["Normal Load", "НАГРУЗКА"], ["N", "Н"], ["Temperature ( Deg C)", "ТЕМПЕРАТУРА (Град С)"], ["Heater On", "НАГРЕВ ВКЛ"], ["Humidity", "ВЛАЖНОСТЬ"], ["Rh", "%"], ["OFF", "ВЫКЛ"], ["Timer", "ВРЕМЯ"], ["Test duration", "ВРЕМЯ ТЕСТА"], ["min", "мин"], ["Elapsed Time", "依商判"], ["Save Dwell", "ИНТЕРВАЛ"], ["Sec", "Сек"], ["Count down ( Sec )", "До запуска (сек)"], ["Present ( Sec )", "Таймер (сек)"], ["Run", "Применить"], ["Power", "ПИТАНИЕ"], ["Test Status", "СТАТУС"], ["Manual Over Ride", "ПУСК"], ["Coefficient Of Friction", "КОЭФФИЦИЕНТ ТРЕНИЯ"], ["Data points", "Точки"], ["Reset Graph", "Сбросить график"], ["Frictional Force ( N )", "СИЛА ТРЕНИЯ (Н)"], ["ISO : WS1.4", "ISO : WS1.4"], ["Rh Before", "Влажность до"], ["Rh After", "Влажность, после"], ["Humidity, before test", "Влажность, до теста"], ["Humidity, after test", "Влажность, после теста"], ["Temp, before test", "Температура, до теста"], ["Temp, after test", "Температура, после теста"], ["AVP ", "СДП"], ["MWSD", "MWSD"], ["HCF", "ФКВ"], ["WS1.4", "WS1.4"], ["Save Result", "Сохранить результат"], ["COMPARE FILES", ""], ["File 1", "ФАЙЛ 1"], ["File 2", "ФАЙЛ 2"], ["File 3", "ФАЙЛ 3"], ["File 4", "ФАЙЛ 4"], ["Refresh", "ОБНОВИТЬ"], ["Coefficient Of Friction", "КОЭФФИЦИЕНТ ТРЕНИЯ"], ["Temperature", "ТЕМПЕРАТУРА"], ["Frictional Force ( N )", "СИЛА ТРЕНИЯ (Н)"], ["COF1", "КОФ1"], ["COF2", "КОФ2"], ["COF3", "КОФ3"], ["COF4", "КОФ4"], ["Reset Graph", "Сбросить график"], ["Time ( mins )", "Время (мин)"], ["Temperature ( Deg C)", "ТЕМПЕРАТУРА (Град С)"], ["Frictional  Force ( N )", "СИЛА ТРЕНИЯ (Н)"], ["ABOUT", ""], ["Frictional Force :", "КОЭФ.ТРЕНИЯ:"], ["Temperature :", "ТЕМПЕРАТУРА"], ["Speed Out:", "СКОРОСТЬ"], ["Air Temperature :", "ТЕМПЕРАТУРА ВОЗДУХА"], ["Humidity :", "ВЛАЖНОСТЬ"], ["Edit Gain Constant", "КОРРЕКТИРОВКА КОНСТАНТ"], ["Save Gain Constant", "СОХРАНИТЬ КОНСТАНТЫ"], ["Calibrate Parameter", "ПАРАМЕТРЫ КАЛИБРОВКИ"], ["Frictional Force ( N )", "СИЛА ТРЕНИЯ (Н)"], ["WINDUCOM 2010 \\XXXX\\VX.XX\\MONTH YEAR", "WINDUCOM 2010 \\XXXX\\VX.XX\\MONTH YEAR"], ["Stroke", "ДЛИННА ХОДА"], ["mm", "мм"], ["Air Temperature", "ВОЗДУХА ТЕМП"], ["Stroke", "ДЛИННА ХОДА "], ["Time ( mins )", "ВРЕМЯ ( мин )"], ["Sample Temperature( Deg C)", "Образец ТЕМПЕРАТУРА (Град С)"], ["Relative Humidity ( Rh )", "Относительный Влажность ( % )"], ["Air Temperature ( deg C )", "ТЕМПЕРАТУРА ВОЗДУХА (Град С)"], ["Save Gain Constants", "СОХРАНИТЬ КОНСТАНТЫ"], ["Password", "ПАРОЛЬ ДОСТУПА"], ["Enter Current Password", "ВВЕДИТЕ ТЕКУЩИЙ ПАРОЛЬ"], ["Enter The New Password", "ВВЕДИТЕ НОВЫЙ ПАРОЛЬ"], ["Change Calibrate Password", "Сбросить пароль калибровки"], ["Newtons ( N )", "Ньютон ( Н )"], ["File path", "Путь к файлу"], ["Threshold", "порог"], ["Run", "ПУСК"], ["Stop", "СТОП"], ["Displacement :", "смещение:"], ["Stroke Gain :", "ДЛИННА ХОДА:"], ["Port 1", "порт 1"], ["Port 2", "порт 2"], ["Ch-Power +:", "CH-ПИТАНИЕ +:"], ["Ch-Power -:", "CH-ПИТАНИЕ -:"], ["Ch-Heater:", "НАГРЕВ:"], ["Ch-Humidity Wet:", "CH-Увлажнение:"], ["Ch-Humidity Dry:", "CH-Осушение:"], ["Heater On", "НАГРЕВ ВКЛ"], ["Heater Off", "НАГРЕВ ВЫКЛ"], ["On", "ВКЛ"], ["Off", "ВЫКЛ"], ["TEXT REPORT", "ПРОТОКОЛ ИСПЫТАНИЯ"], ["Open Data File", "ОТКРЫТЬ ФАЙЛ ДАННЫХ"], ["Refresh", "ОБНОВЛЕНО"], ["Tittle", "заглавие"], ["Sample Design", "Образец"], ["Tested date", "Дата"], ["Sample ID ", "Имя образца"], ["Tested by", "Испытано"], ["System Configured Printers ", "Сконфигурированные принтеры"], ["Selected Printer", "Выбранный принтер"], ["Select Printer 3", "Выбрать  Печать"], ["Print", "Печать"], [":-@(WINDUCOM : RECIPROCATORY TEST RIG    DEFINITON FILE )      ", "(Анализатор HFRR с возвратно-поступательным механизмом для определения смазывающей способности дизельных топлив )"], ["Tested by:", "Оператор:"], ["          TIME;      COF;       STROKE  (mm);     AIR TEMP ( Deg C);  TEMP ( Deg C);  HUMIDITY ( Rh );", "КОЭФФИЦИЕНТ ТРЕНИЯ;   Инсульт; ТЕМПЕРАТУРА ВОЗДУХА; ВЛАЖНОСТЬ;"], ["Export", "Экспорт"], ["Temperature Intercept :", "ТЕМП перехват:"], ["Air Temperature Intercept:", "ТЕМП  ВОЗДУХА перехват:"], ["Select File Type ", "Выберете формат файла"], ["S.NO", "S.NO"], ["Trip", ""]]
  out "Fric Val":dbl[](array[numeric])
